vi "Write Result.vi"(0 "Scalar Charact Result Accessor in":refnum<class "Scalar Charact Result Accessor.lvclass">, 5 "Charact Result":variant, 11 "error in":errorcluster) -> (4 "Scalar Charact Result Accessor out":refnum<class "Scalar Charact Result Accessor.lvclass">, 15 "error out":errorcluster)   [LabVIEW 2023, in "RFFixtureCharact.Public.lvlib" / "Scalar Charact Result Accessor.lvclass"]
uses:
  Scalar Charact Result Accessor.lvclass
  C:/rfcal/AuxTools/STSRFFixtureCharactUtility/Source/Code Modules/Fixture/RMM/Charact Result Accessor/Base/Charact Result Accessor.lvclass
  Base Classes/Scalar/Scalar Path/Type Definitions/Scalar Charact Result.ctl
  <vilib>/addons/_RFCalAndCharactDatabase/NI_RFCalAndCharact_Database_API.lvlibp/Characterization/Controls/Type.ctl
  Scalar Charact Result Accessor.lvclass/Scalar Charact Result Accessor.ctl
  Base Classes/Scalar/Scalar Path/Scalar Path.lvclass
  <vilib>/addons/_RFCalAndCharactDatabase/NI_RFCalAndCharact_Database_API.lvlibp/Characterization/Characterization.lvlib
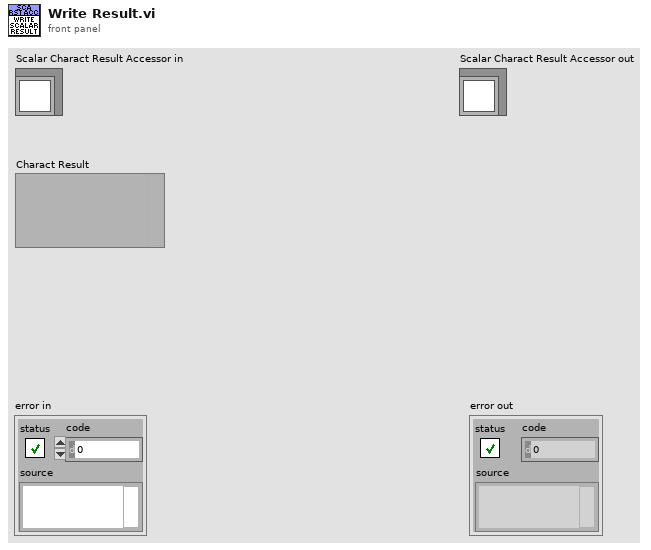
[diagram p1: front panel]
types:
  T1 = typedef "RFFixtureCharact.Public.lvlib/Scalar Path.lvclass/Scalar Charact Result.ctl" = cluster{"Port Power":dbl, "Reference Level":dbl, "Frequency":dbl, "Path Gain":dbl, "Out Of Limit":bool}
  T2 = typedef "NI_RFCalAndCharact_Database_API.lvlibp/Characterization.lvlib/Type.ctl" = u16
  T3 = typedef "NI_RFCalAndCharact_Database_API.lvlibp/Characterization.lvlib/Path Handle.ctl" = refnum<k24>
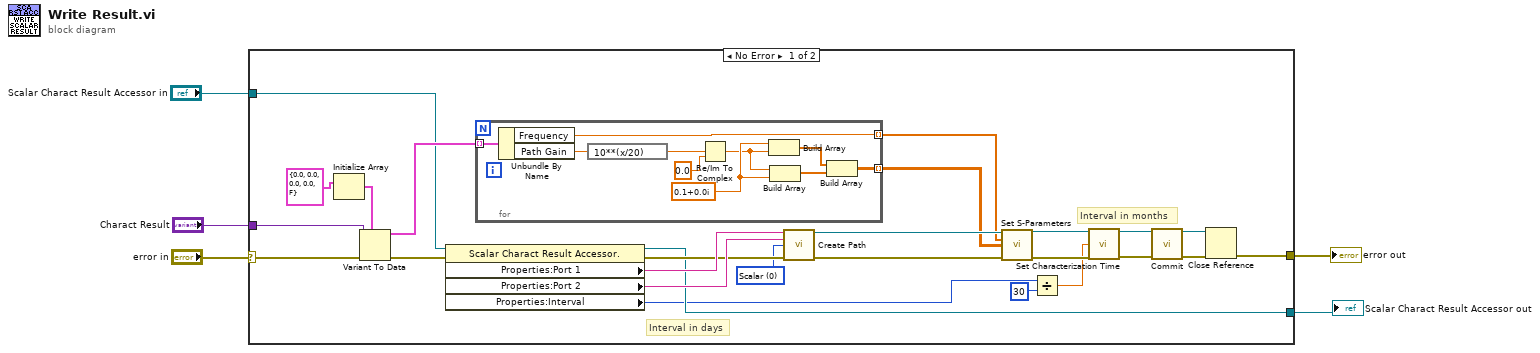
[diagram p0: block diagram]
diagram:
  n1 = case shown="No Error" "error in" {
    selector: "error in" -> [w29 w43]
    tunnel: [w10 w43] -> w1
    tunnel: "Charact Result" -> [w28 _]
    tunnel: "Scalar Charact Result Accessor in" -> [w25 w42]
    tunnel: [w9 w42] -> w2
    frame No Error {
      w21 = T2 0 items=["Scalar", "Vector"] ("Type")
      # "Interval in months"
      # "Interval in days"
      n2 = Initialize Array(T1 {"Port Power"=0.0, "Reference Level"=0.0, "Frequency"=0.0, "Path Gain"=0.0, "Out Of Limit"=FALSE} ("Charact Result")) -> (w30:T1[])  [unwired: 1 in]
      n3 = Variant To Data(error in=w29, type=w30, Variant=w28) -> (data=w27:T1[], error out=w26:errorcluster)
      n4 = property class="Scalar Charact Result Accessor."(reference=w25, error in=w26) -> (reference out=w9:refnum<class "Scalar Charact Result Accessor.lvclass">, error out=w22:errorcluster, "Properties:Port 1"=w24:string, "Properties:Port 2"=w23:string, "Properties:Interval"=w8:i32)
      n5 = for {
        tunnel: w27 -> [w41] mode=indexing
        tunnel: [w40] -> w16 mode=indexing
        tunnel: [w32] -> w15 mode=indexing
        w36 = cdb 0.1+0.0i ("element")
        n6 = Unbundle By Name(w41) -> ("Frequency"=w40:dbl, "Path Gain"=w38:dbl)
        n7 = expression code="10**(x/20)"(w38) -> (w37:dbl)
        n8 = Re/Im To Complex(1:0.0 ("y"), 2:w37) -> (0:w35:cdb)
        n9 = Build Array(w36, w35) -> (w34:cdb[])
        n10 = Build Array(w35, w36) -> (w33:cdb[])
        n11 = Build Array(w34, w33) -> (w32:cdb[][])
      }
      n12 = call <vilib>:"Create Path.vi"("Port 1"=w24, "Port 2"=w23, "Type"=w21, "error in"=w22) -> ("Path"=w17:T3, "error out"=w20:errorcluster)  [unwired: 10 in]
      n13 = call <vilib>:"Set S-Parameters.vi"("Path In"=w17, "Frequencies (Hz)"=w16, "S-Parameters"=w15, "error in"=w20) -> ("Path Out"=w18:T3, "error out"=w19:errorcluster)  [unwired: 10 in]
      n14 = Divide(x=w8, y=30) -> (x/y=w6:dbl)
      n15 = call <vilib>:"Set Characterization Time.vi"("Path In"=w18, "Interval (Months)"=w6, "error in"=w19) -> ("Path Out"=w13:T3, "error out"=w14:errorcluster)  [unwired: 11 in]
      n16 = call <vilib>:"Commit.vi"("Path In"=w13, "error in"=w14) -> ("Path Out"=w11:T3, "error out"=w12:errorcluster)  [unwired: 12 in]
      n17 = Close Reference(reference=w11, error in (no error)=w12) -> (error out=w10:errorcluster)
    }
    frame Error {
    }
  }
  "error out" <- w1
  "Scalar Charact Result Accessor out" <- w2
